vi "A33ConfigureRamp.vi"(8 "error in (no error)":errorcluster, 9 "Ramp symmetry (50%)":dbl=50.0 format="%#_12g", 10 "Channel (1: Channel1)":u16(ring)=1 items=["Channel1"=1, "Channel2"=2], 11 "VISA resource name":refnum<visa-resource-name>) -> (0 "error out":errorcluster, 3 "VISA resource name out":refnum<visa-resource-name>)   [LabVIEW 2022 SP3]
doc: "Selects the waveform shape, frequency, amplitude, offset, and phase for a standard waveform."
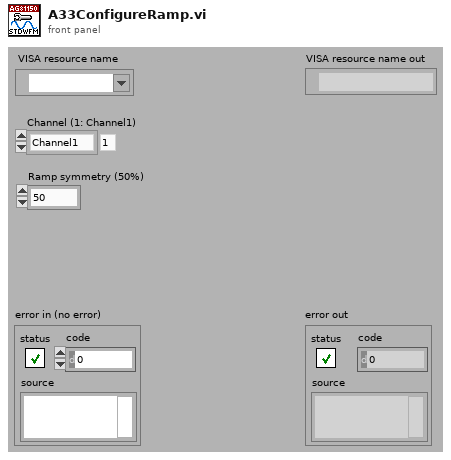
[diagram p1: front panel]
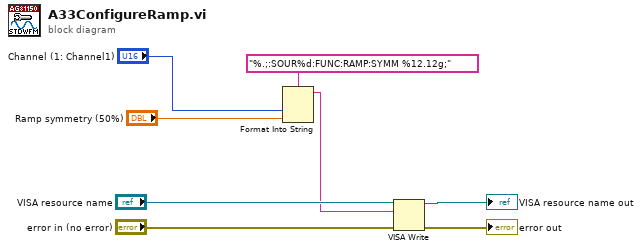
[diagram p0: block diagram]
diagram:
  n1 = Format Into String(format string="%.;:SOUR%d:FUNC:RAMP:SYMM %12.12g;", "Channel (1: Channel1)", "Ramp symmetry (50%)") -> (resulting string=w1:string)  [unwired: 2 in, 1 out]
  n2 = VISA Write(VISA resource name="VISA resource name", write buffer=w1, error in (no error)="error in (no error)") -> (VISA resource name out=→"VISA resource name out":refnum<visa-resource-name>, error out=→"error out":errorcluster)  [unwired: 1 out]
